vi "Edit_Raw_DF.vi"(5 "Edit Raw Data Header Info":bool, 6 "New Analysis Info Cluster Setup":string, 7 "New Values In":string[](array[string])=[""], 8 "New Chs In":string[](array[string])=[""], 9 "Data filename":path) -> (0 "Filetype":string, 1 "Original values":string[](array[string]), 3 "Data filename out":path, 4 "File Not Changed?":bool)   [LabVIEW 2020]
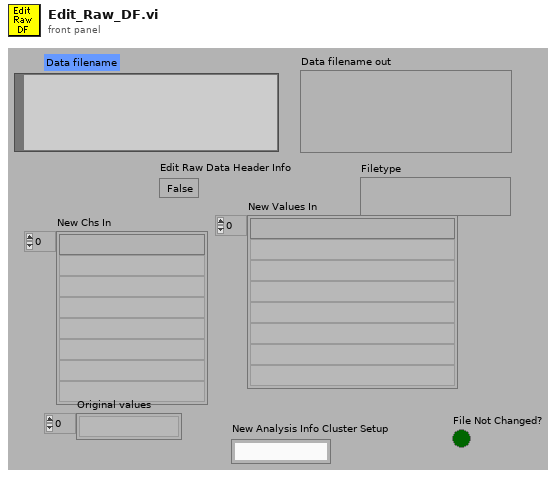
[diagram p1: front panel]
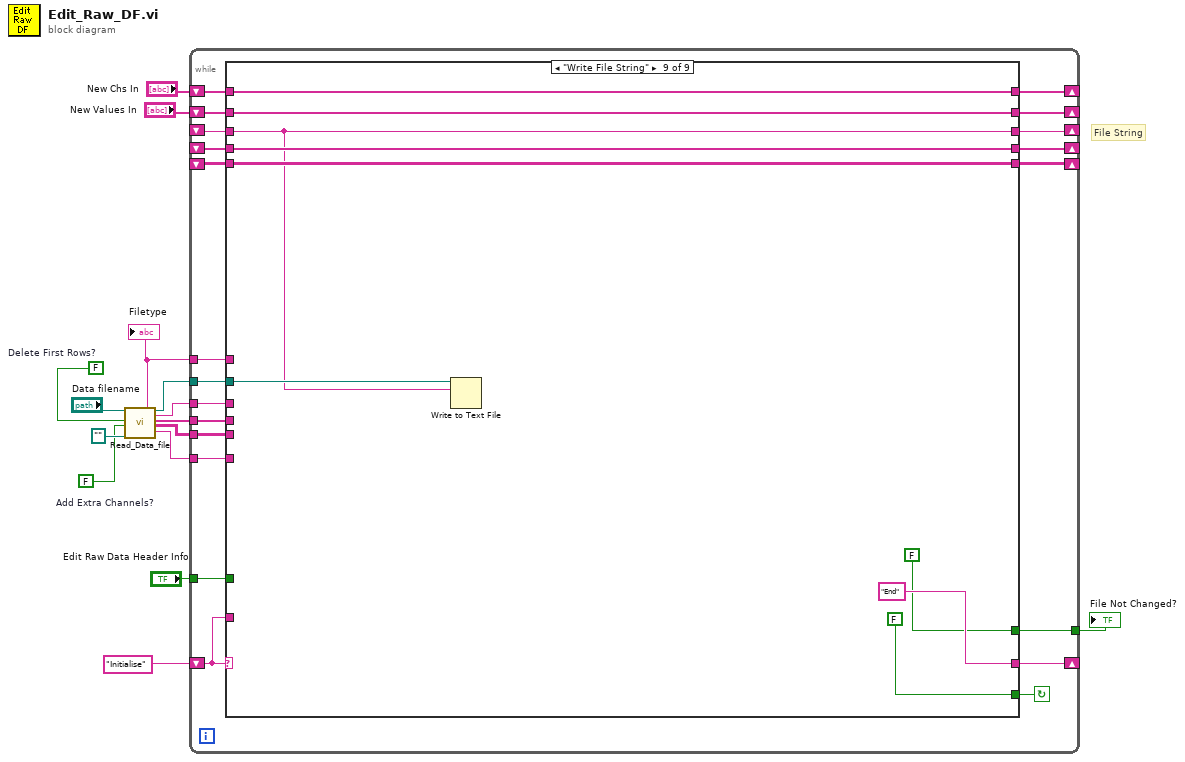
[diagram p0: block diagram]
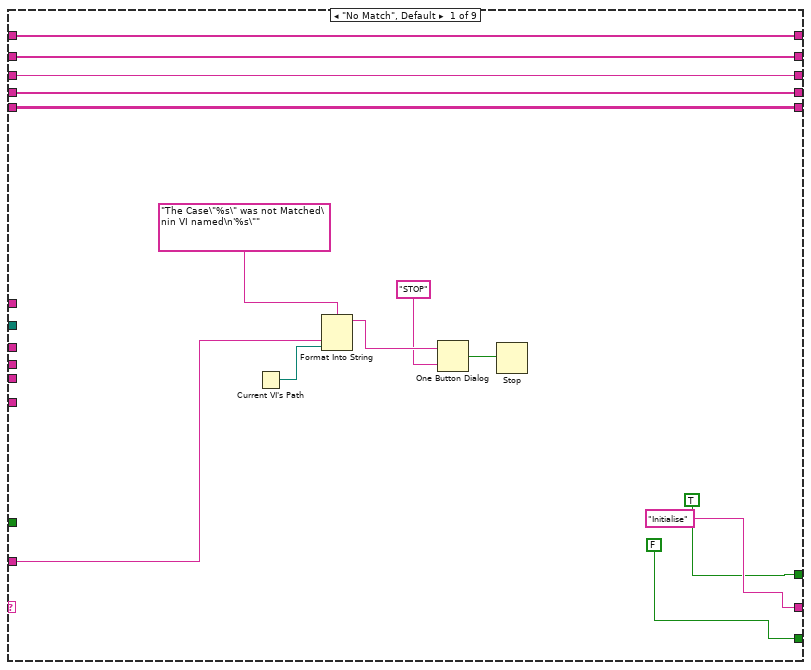
[diagram p2: hidden frame]
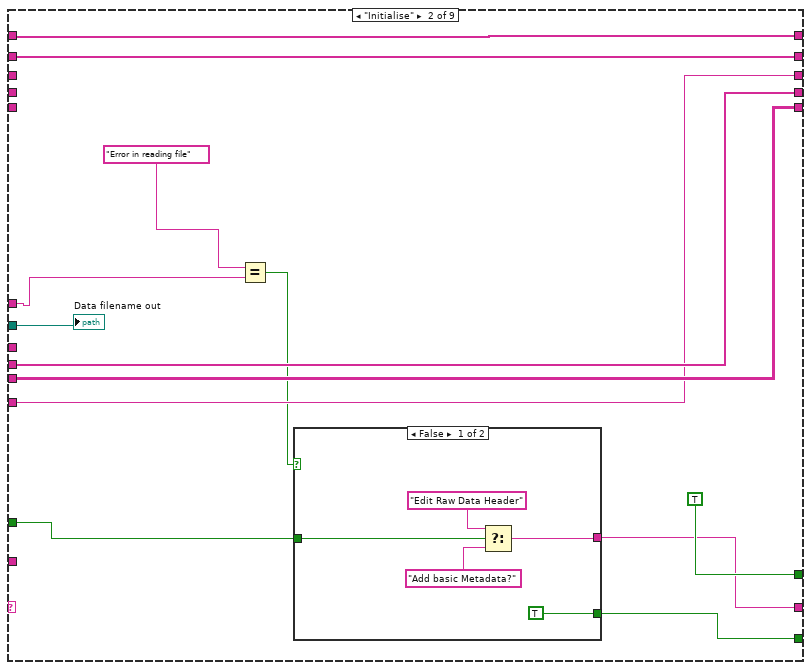
[diagram p3: hidden frame]
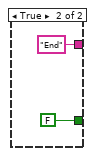
[diagram p4: hidden frame]
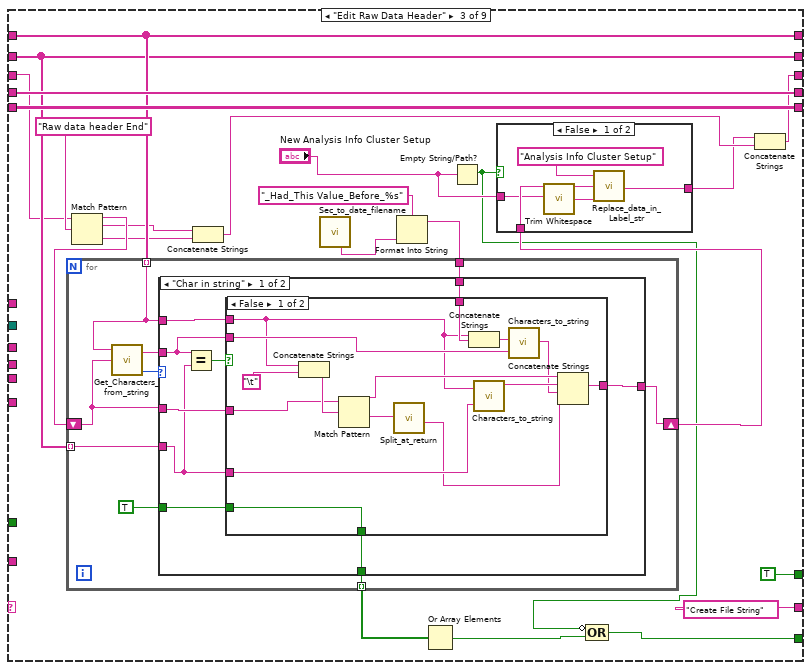
[diagram p5: hidden frame]
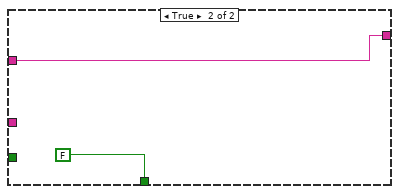
[diagram p7: hidden frame]
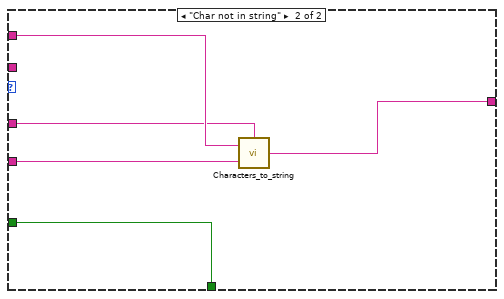
[diagram p8: hidden frame]
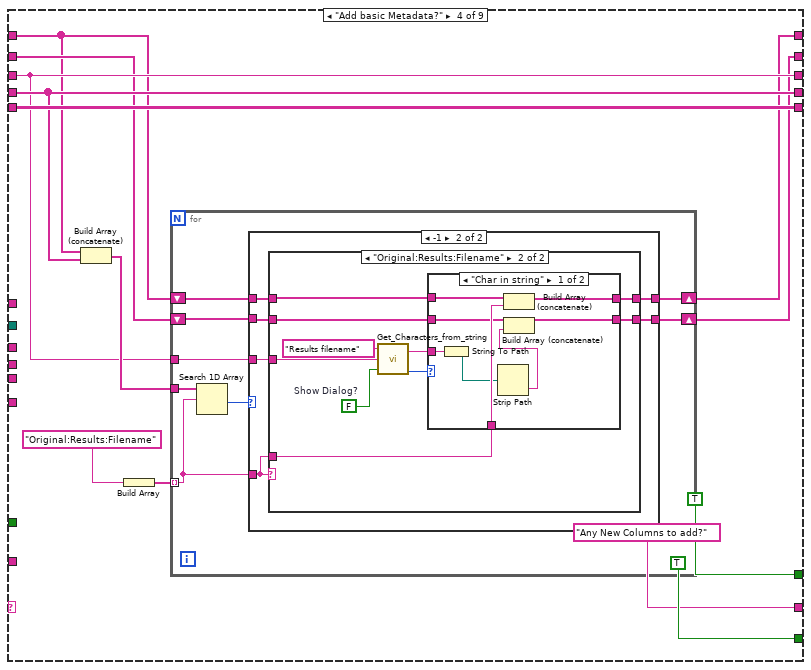
[diagram p9: hidden frame]
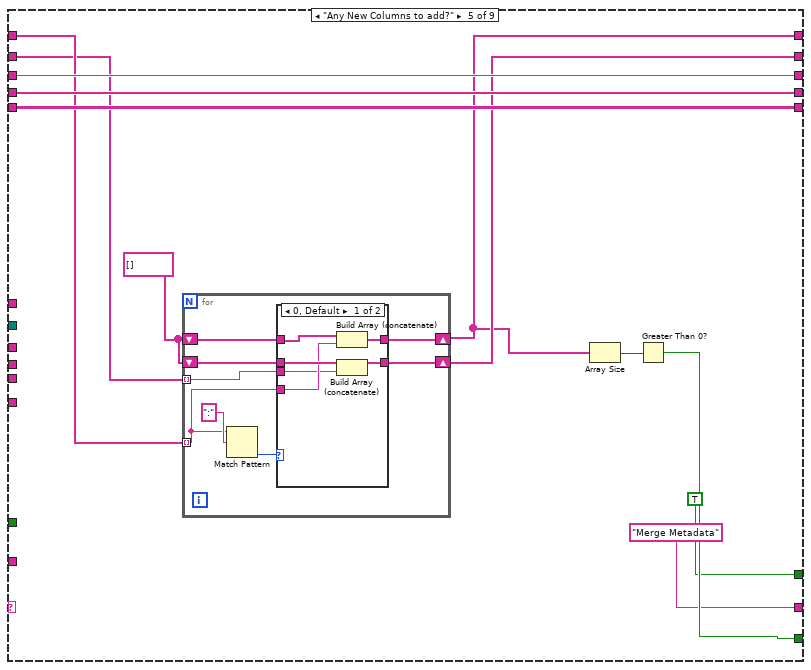
[diagram p13: hidden frame]
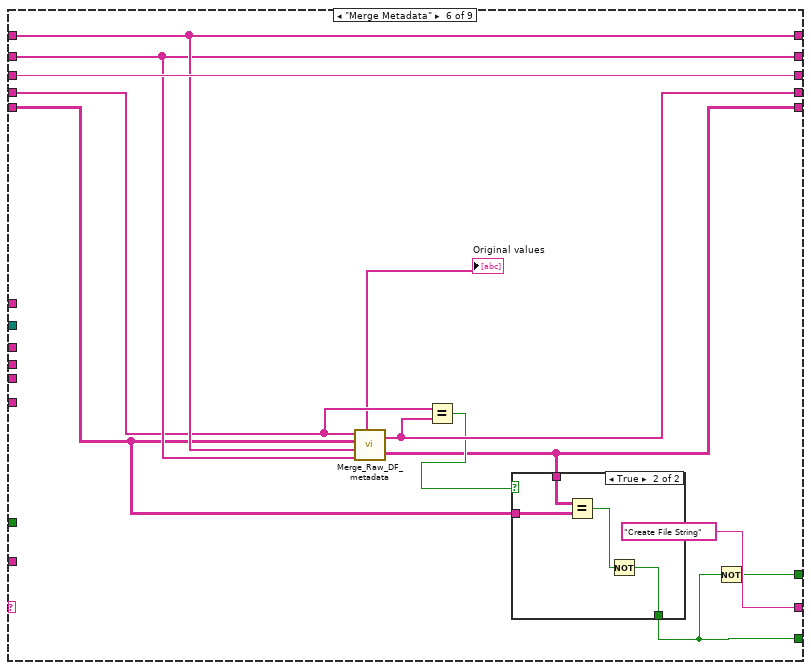
[diagram p15: hidden frame]
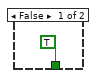
[diagram p16: hidden frame]
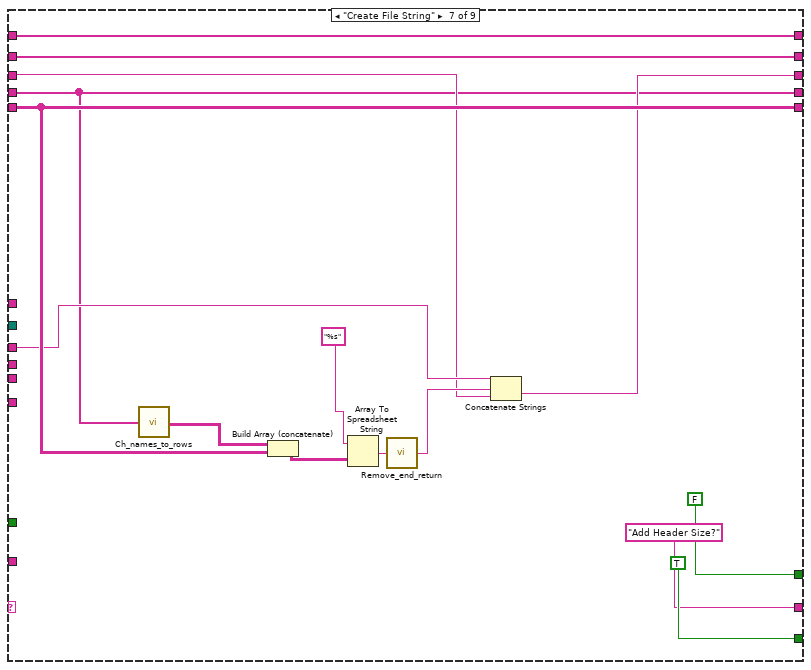
[diagram p17: hidden frame]
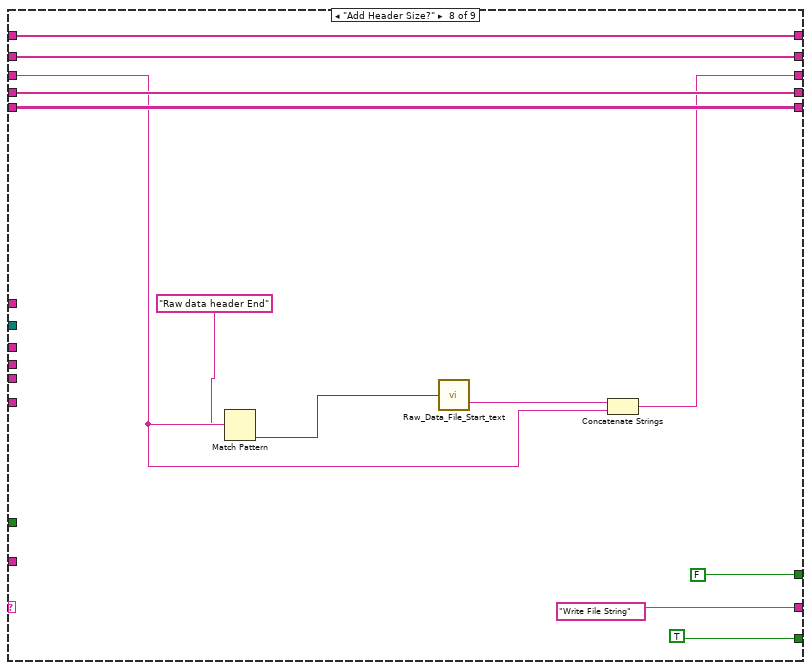
[diagram p18: hidden frame]
diagram:
  w1 = FALSE  # Delete First Rows?
  w13 = FALSE  # Add Extra Channels?
  # "File String"
  n1 = call "Read_Data_file.vi"("Results file"="Data filename", "Delete First Rows?"=w1, "Add Extra Channels?"=w13, "Template File"=path "") -> ("Filetype"=w8:string, "Results file Out"=w11:path, "String Before"=w7:string, "Ch names Out"=w10:string[], "Channel Values Out"=w9:string[][], "String After"=w6:string)  [unwired: 3 in, 7 out]
  "Filetype" <- w8
  n2 = while {
    tunnel: "Edit Raw Data Header Info" -> [w17]
    shift-left: "New Values In" -> [w19]
    shift-right: [w18] -> _
    shift-left: "New Chs In" -> [w21]
    shift-right: [w20] -> _
    tunnel: w6 -> [w22]
    tunnel: w7 -> [w23]
    tunnel: w8 -> [w24]
    tunnel: w9 -> [w25]
    tunnel: w10 -> [w26]
    tunnel: w11 -> [w27]
    shift-left: _ -> [w28]
    shift-right: [w32] -> _
    shift-left: _ -> [w29]
    shift-right: [w31] -> _
    shift-left: _ -> [w30]
    shift-right: [w33] -> _
    shift-left: "Initialise" -> [w34]
    shift-right: [w35] -> _
    tunnel: [w16] -> w2
    stop <- w36 continue-if-true
    n3 = case shown="\"Write File String\"" w34 {
      tunnel: [FALSE w51 w72 TRUE w198 w221 TRUE TRUE FALSE] -> w36
      tunnel: ["Initialise" w55 "Create File String" ("f") "Any New Columns to add?" "Merge Metadata" ("f") "Create File String" ("f") "Add Header Size?" ("f") "Write File String" "End"] -> w35
      tunnel: w34 -> [w45 _ _ _ _ _ _ _ _]
      tunnel: [w42 w58 w80 w145 w202 w230 w243 w258 w263] -> w33
      tunnel: [w40 w59 w93 w151 w201 w224 w245 w260 w269] -> w32
      tunnel: [w41 w60 w92 w148 w200 w227 w237 w261 w270] -> w31
      tunnel: w30 -> [w42 _ w85 w145 w202 w230 w239 w259 w263]
      tunnel: w29 -> [w41 _ w92 w148 w200 w226 w237 w261 w270]
      tunnel: w28 -> [w40 _ w93 w151 w201 w223 w245 w260 w269]
      tunnel: w27 -> [_ w63 _ _ _ _ _ _ w264]
      tunnel: w26 -> [_ w60 _ _ _ _ _ _ _]
      tunnel: w25 -> [_ w59 _ _ _ _ _ _ _]
      tunnel: w24 -> [_ w53 _ _ _ _ _ _ _]
      tunnel: w23 -> [_ _ _ _ _ _ w244 _ _]
      tunnel: w22 -> [_ w58 _ _ _ _ _ _ _]
      tunnel: w21 -> [w39 w62 w88 w141 w194 w229 w241 w257 w267]
      tunnel: [w39 w62 w88 w144 w192 w229 w241 w257 w267] -> w20
      tunnel: w19 -> [w38 w61 w87 w142 w193 w228 w240 w256 w266]
      tunnel: [w38 w61 w87 w143 w195 w228 w240 w256 w266] -> w18
      tunnel: w17 -> [_ w56 _ _ _ _ _ _ _]
      tunnel: [TRUE TRUE TRUE TRUE TRUE w220 FALSE FALSE FALSE] -> w16
      frame "No Match", Default {
        n4 = Current VI's Path() -> (path=w44:path)
        n5 = Format Into String(format string="The Case\"%s\" was not Matched\nin VI named\n'%s\"" ("Format String"), w45, w44) -> (resulting string=w48:string)  [unwired: 2 in, 1 out]
        n6 = One Button Dialog(message=w48, button name ("OK")="STOP") -> (true=w46:bool)
        n7 = Stop(stop? (T)=w46) -> ()
      }
      frame "Initialise" {
        n8 = Equal?(x="Error in reading file", y=w53) -> (x = y?=w52:bool)
        n9 = case shown="False" w52 {
          tunnel: w56 -> [w66 _]
          tunnel: [w65 "End"] -> w55
          tunnel: [TRUE FALSE] -> w51
          frame False {
            n10 = Select(t="Edit Raw Data Header", s=w66, f="Add basic Metadata?") -> (s? t:f=w65:string)
          }
          frame True {
          }
        }
        "Data filename out" <- w63
      }
      frame "Edit Raw Data Header" {
        n11 = Match Pattern(string=w85, regular expression="Raw data header End") -> (before substring=w84:string, match substring=w83:string, after substring=w82:string)  [unwired: 2 out]
        n12 = Concatenate Strings(w83, w82) -> (w81:string)
        n13 = call "Sec_to_date_filename.vi"() -> ("YYYY-mm-DD HH:MM"=w77:string)  [unwired: 6 in, 9 out]
        n14 = Format Into String(format string="_Had_This Value_Before_%s" ("Format String"), w77) -> (resulting string=w90:string)  [unwired: 2 in, 1 out]
        n15 = for {
          shift-right: [w103] -> w76
          shift-left: w84 -> [w105]
          tunnel: w88 -> [w106] mode=indexing
          tunnel: w87 -> [w104] mode=indexing
          tunnel: w90 -> [w102]
          tunnel: [w101] -> w78 mode=indexing
          n16 = call "Get_Characters_from_string.vi"("Input string"=w105, "Variable name"=w106) -> ("Status"=w108:enum16{"Char in string", "Char not in string"}, "Value"=w107:string)  [unwired: 1 in]
          n17 = case shown="\"Char in string\"" w108 {
            tunnel: w106 -> [w115 w139]
            tunnel: w104 -> [w114 w138]
            tunnel: [w116 w135] -> w103
            tunnel: w105 -> [w117 w136]
            tunnel: w107 -> [w112 _]
            tunnel: w102 -> [w111 _]
            tunnel: [w110 w137] -> w101
            tunnel: TRUE -> [w109 w137]
            frame "Char in string" {
              n18 = Equal?(x=w112, y=w114) -> (x = y?=w113:bool)
              n19 = case shown="False" w113 {
                tunnel: w117 -> [w130 w134]
                tunnel: [w128 w134] -> w116
                tunnel: w114 -> [w127 _]
                tunnel: w115 -> [w121 _]
                tunnel: w112 -> [w123 _]
                tunnel: w111 -> [w122 _]
                tunnel: [w118 FALSE] -> w110
                tunnel: w109 -> [w118 _]
                frame False {
                  n20 = Concatenate Strings(w121, "\t") -> (w131:string)
                  n21 = Match Pattern(string=w130, regular expression=w131) -> (before substring=w125:string, after substring=w129:string)  [unwired: 3 out]
                  n22 = call "Split_at_return.vi"("String"=w129) -> ("after substring"=w124:string)  [unwired: 1 in, 3 out]
                  n23 = Concatenate Strings(w121, w122) -> (w120:string)
                  n24 = call "Characters_to_string.vi"("Characters to write"=w127, "Label for characters"=w121) -> ("Output string"=w126:string)  [unwired: 1 in]
                  n25 = call "Characters_to_string.vi"("Characters to write"=w123, "Label for characters"=w120) -> ("Output string"=w119:string)  [unwired: 1 in]
                  n26 = Concatenate Strings(w125, w126, w119, w124) -> (w128:string)
                }
                frame True {
                }
              }
            }
            frame "Char not in string" {
              n27 = call "Characters_to_string.vi"("stringIn"=w136, "Characters to write"=w138, "Label for characters"=w139) -> ("Output string"=w135:string)
            }
          }
        }
        n28 = Or Array Elements(Boolean array=w78) -> (logical OR=w73:bool)
        n29 = Empty String/Path?(string/path="New Analysis Info Cluster Setup") -> (empty?=w71:bool)
        n30 = case shown="False" w71 {
          tunnel: w76 -> [w96 w99]
          tunnel: [w97 w99] -> w75
          tunnel: "New Analysis Info Cluster Setup" -> [w95 _]
          frame False {
            n31 = call <vilib>:"Trim Whitespace.vi"("string"=w95) -> ("trimmed string"=w94:string)  [unwired: 1 in]
            n32 = call "Replace_data_in_Label_str.vi"("New data string"=w94, "Input string"=w96, "Variable name"="Analysis Info Cluster Setup") -> ("Appended string"=w97:string)
          }
          frame True {
          }
        }
        n33 = Compound Arithmetic op=OR(invert w71, w73) -> (w72:bool)
        n34 = Concatenate Strings(w75, w81) -> (w80:string)
      }
      frame "Add basic Metadata?" {
        n35 = Build Array (concatenate)(w141, w148) -> (w146:string[])
        n36 = Build Array("Original:Results:Filename") -> (w147:string[])
        n37 = for {
          tunnel: w147 -> [w158] mode=indexing
          tunnel: w146 -> [w159]
          shift-right: [w157] -> w144
          shift-left: w141 -> [w156]
          shift-right: [w154] -> w143
          shift-left: w142 -> [w155]
          tunnel: w145 -> [w153]
          n38 = Search 1D Array(1D array=w159, element=w158) -> (index of element=w160:i32)  [unwired: 1 out]
          n39 = case shown="-1" w160 {
            tunnel: w158 -> [_ w163]
            tunnel: [w162 w168] -> w157
            tunnel: w156 -> [w162 w167]
            tunnel: w155 -> [w161 w166]
            tunnel: [w161 w165] -> w154
            tunnel: w153 -> [_ w164]
            frame 0, Default {
            }
            frame -1 {
              n40 = case shown="\"Original:Results:Filename\"" w163 {
                tunnel: [w170 w174] -> w168
                tunnel: w167 -> [w170 w176]
                tunnel: w166 -> [w169 w172]
                tunnel: [w169 w171] -> w165
                tunnel: w164 -> [_ w179]
                tunnel: w163 -> [_ w175]
                frame "Other", Default {
                }
                frame "Original:Results:Filename" {
                  w178 = FALSE  # Show Dialog?
                  n41 = call "Get_Characters_from_string.vi"("Show Dialog?"=w178, "Input string"=w179, "Variable name"="Results filename") -> ("Status"=w177:enum16{"Char in string", "Char not in string"}, "Value"=w173:string)
                  n42 = case shown="\"Char in string\"" w177 {
                    tunnel: w176 -> [w188 w190]
                    tunnel: w175 -> [w187 _]
                    tunnel: [w186 w190] -> w174
                    tunnel: w173 -> [w185 _]
                    tunnel: w172 -> [w183 w189]
                    tunnel: [w182 w189] -> w171
                    frame "Char in string" {
                      n43 = String To Path(string=w185) -> (path=w184:path)
                      n44 = Strip Path(path=w184) -> (name=w181:string)  [unwired: 1 out]
                      n45 = Build Array (concatenate)(w188, w187) -> (w186:string[])
                      n46 = Build Array (concatenate)(w183, w181) -> (w182:string[])
                    }
                    frame "Char not in string" {
                    }
                  }
                }
              }
            }
          }
        }
      }
      frame "Any New Columns to add?" {
        w196 = string[] []
        n47 = for {
          tunnel: w194 -> [w204] mode=indexing
          shift-right: [w205] -> w192
          shift-left: w196 -> [w208]
          shift-right: [w207] -> w195
          shift-left: w196 -> [w206]
          tunnel: w193 -> [w203] mode=indexing
          n48 = Match Pattern(string=w204, regular expression=":") -> (offset past match=w209:i32)  [unwired: 4 out]
          n49 = case shown="0, Default" w209 {
            tunnel: [w213 w218] -> w205
            tunnel: w208 -> [w216 w218]
            tunnel: [w214 w217] -> w207
            tunnel: w206 -> [w215 w217]
            tunnel: w204 -> [w212 _]
            tunnel: w203 -> [w211 _]
            frame 0, Default {
              n50 = Build Array (concatenate)(w216, w212) -> (w213:string[])
              n51 = Build Array (concatenate)(w215, w211) -> (w214:string[])
            }
            frame -1 {
            }
          }
        }
        n52 = Array Size(array=w192) -> (size(s)=w199:i32)
        n53 = Greater Than 0?(x=w199) -> (x > 0?=w198:bool)
      }
      frame "Merge Metadata" {
        n54 = call "Merge_Raw_DF_metadata.vi"("New Values In"=w228, "New Chs In"=w229, "Orig Values In"=w223, "Orig Chs In"=w226) -> ("Channel Values Out"=w224:string[][], "Ch names Out"=w227:string[], "Original values"=→"Original values":string[])  [unwired: 1 in]
        n55 = Equal?(x=w226, y=w227) -> (x = y?=w225:bool)
        n56 = case shown="True" w225 {
          tunnel: [TRUE w232] -> w221
          tunnel: w224 -> [_ w235]
          tunnel: w223 -> [_ w234]
          frame False {
          }
          frame True {
            n57 = Equal?(x=w235, y=w234) -> (x = y?=w233:bool)
            n58 = Not(x=w233) -> (.not. x?=w232:bool)
          }
        }
        n59 = Not(x=w221) -> (.not. x?=w220:bool)
      }
      frame "Create File String" {
        n60 = call "Ch_names_to_rows.vi"("Channel Names"=w237) -> ("3 Row names"=w236:string[][])
        n61 = Build Array (concatenate)(w236, w245) -> (w246:string[][])
        n62 = Array To Spreadsheet String(array=w246, 3:"%s" ("format string")) -> (spreadsheet string=w248:string)  [unwired: 1 out]
        n63 = call "Remove_end_return.vi"("Input string"=w248) -> ("Output string"=w249:string)
        n64 = Concatenate Strings(w244, w249, w239) -> (w243:string)
      }
      frame "Add Header Size?" {
        n65 = Match Pattern(string=w259, regular expression="Raw data header End") -> (offset past match=w253:i32)  [unwired: 4 out]
        n66 = call "Raw_Data_File_Start_text.vi"("Header length"=w253) -> ("Start String"=w252:string)
        n67 = Concatenate Strings(w252, w259) -> (w258:string)
      }
      frame "Write File String" {
        n68 = Write to Text File(file (use dialog)=w264, text=w263) -> ()  [unwired: 2 in, 3 out]
      }
    }
  }
  "File Not Changed?" <- w2
